vi "Terminal Coupling to String.vi"(11 "Coupling":T1 items=[""=0, "AC"=10045, "DC"=10050, "GND"=10066]) -> (3 "String":string)   [LabVIEW 2019, in "Instrument.Lockin.lvlib" / "Instrument.Lockin.lvclass"]
uses:
  Instrument.Lockin.lvclass
  Instrument.DAQ/Typedefs/DAQ.Config.AI.Coupling--enum.ctl
  Instrument.DAQ/Instrument.DAQ.lvclass
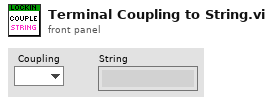
[diagram p1: front panel]
types:
  T1 = typedef "Instrument.Lockin.lvlib/Instrument.DAQ.lvclass/DAQ.Config.AI.Coupling--enum.ctl" = u16
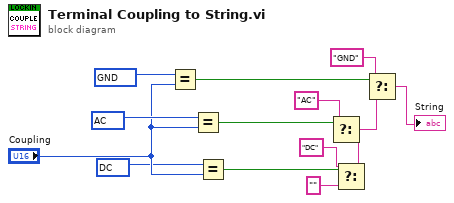
[diagram p0: block diagram]
diagram:
  w4 = T1 10050 items=[""=0, "AC"=10045, "DC"=10050, "GND"=10066] ("Coupling")
  w8 = T1 10045 items=[""=0, "AC"=10045, "DC"=10050, "GND"=10066] ("Coupling")
  w14 = T1 10066 items=[""=0, "AC"=10045, "DC"=10050, "GND"=10066] ("Coupling")
  n1 = Equal?(x=w14, y="Coupling") -> (x = y?=w13:bool)
  n2 = Equal?(x=w8, y="Coupling") -> (x = y?=w9:bool)
  n3 = Equal?(x=w4, y="Coupling") -> (x = y?=w6:bool)
  n4 = Select(t="DC", s=w6, f="") -> (s? t:f=w2:string)
  n5 = Select(t="AC", s=w9, f=w2) -> (s? t:f=w7:string)
  n6 = Select(t="GND", s=w13, f=w7) -> (s? t:f=→"String":string)
